vi "GDSString_ResetTextStyle.vi"(0 "TextIn":refnum<vi>, 1 "Text.Font:Name":string, 2 "Text.Font:Size":u32, 3 "Color Box":u32(colorbox)=16777216, 4 "ResetBold(True)":bool, 5 "error in":errorcluster) -> (14 "TextOut":refnum<vi>, 19 "error out":errorcluster)   [LabVIEW 2014]
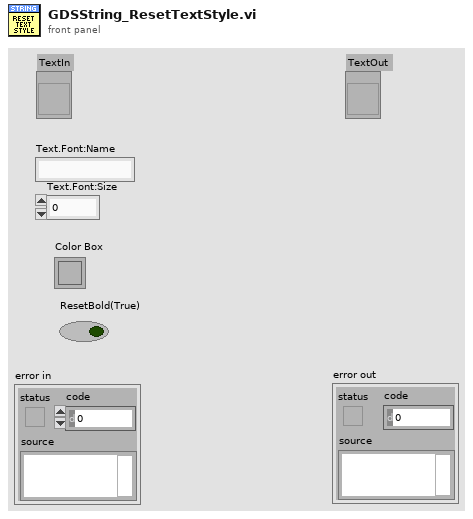
[diagram p1: front panel]
types:
  T1 = cluster{"Selection Start":u32, "Selection End":u32}
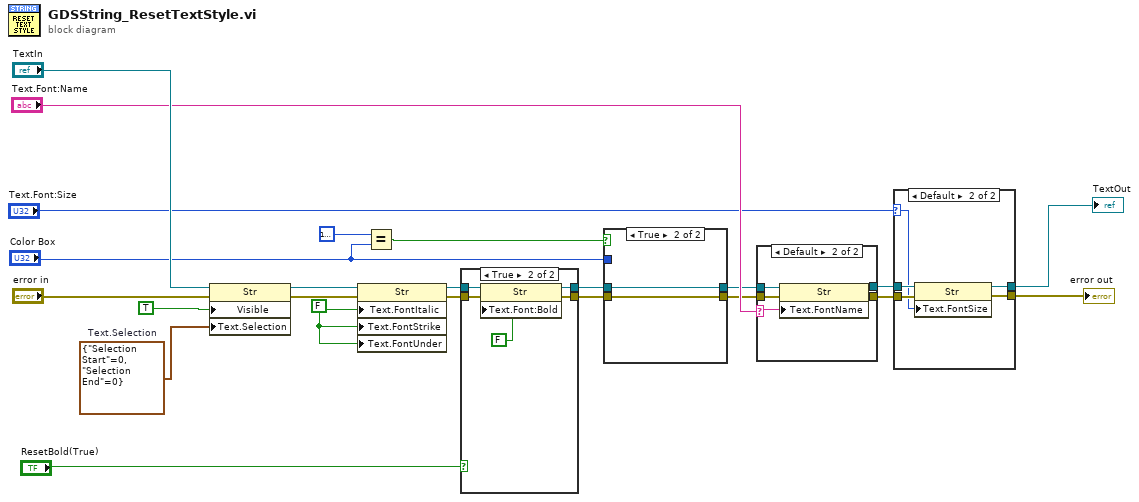
[diagram p0: block diagram]
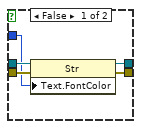
[diagram p3: hidden frame]
diagram:
  w17 = FALSE ("Text.Font:Bold")
  w23 = T1 {"Selection Start"=0, "Selection End"=0}  # Text.Selection
  n1 = property on="Property Node" class="Str"(reference="TextIn", error in="error in", "Visible"=TRUE, "Text.Selection"=w23) -> (reference out=w19:refnum<vi>, error out=w18:errorcluster)
  n2 = property on="Property Node" class="Str"(reference=w19, error in=w18, "Text.FontItalic"=w17, "Text.FontStrike"=w17, "Text.FontUnder"=w17) -> (reference out=w4:refnum<vi>, error out=w3:errorcluster)
  n3 = Equal?(x=u32 16777216 ("Color Box"), y="Color Box") -> (x = y?=w7:bool)
  n4 = case shown="True" "ResetBold(True)" {
    tunnel: w4 -> [w25 w30]
    tunnel: w3 -> [w24 w29]
    tunnel: [w25 w28] -> w2
    tunnel: [w24 w27] -> w1
    frame False {
    }
    frame True {
      n5 = property on="Property Node" class="Str"(reference=w30, error in=w29, "Text.Font:Bold"=FALSE) -> (reference out=w28:refnum<vi>, error out=w27:errorcluster)
    }
  }
  n6 = case shown="True" w7 {
    tunnel: w2 -> [w35 w37]
    tunnel: w1 -> [w34 w36]
    tunnel: [w33 w37] -> w10
    tunnel: [w32 w36] -> w9
    tunnel: "Color Box" -> [w31 _]
    frame False {
      n7 = property on="Property Node" class="Str"(reference=w35, error in=w34, "Text.FontColor"=w31) -> (reference out=w33:refnum<vi>, error out=w32:errorcluster)
    }
    frame True {
    }
  }
  n8 = case shown="Default" "Text.Font:Name" {
    selector: "Text.Font:Name" -> [_ w40]
    tunnel: w10 -> [w39 w44]
    tunnel: w9 -> [w38 w43]
    tunnel: [w39 w42] -> w16
    tunnel: [w38 w41] -> w15
    frame "" {
    }
    frame Default {
      n9 = property on="Property Node" class="Str"(reference=w44, error in=w43, "Text.FontName"=w40) -> (reference out=w42:refnum<vi>, error out=w41:errorcluster)
    }
  }
  n10 = case shown="Default" "Text.Font:Size" {
    selector: "Text.Font:Size" -> [_ w47]
    tunnel: w16 -> [w46 w51]
    tunnel: w15 -> [w45 w50]
    tunnel: [w45 w49] -> w14
    tunnel: [w46 w48] -> w13
    frame 0 {
    }
    frame Default {
      n11 = property on="Property Node" class="Str"(reference=w51, error in=w50, "Text.FontSize"=w47) -> (reference out=w48:refnum<vi>, error out=w49:errorcluster)
    }
  }
  "error out" <- w14
  "TextOut" <- w13
